vi "Save Icon.vi"(8 "error in (no error)":errorcluster, 10 "path":path, 11 "vi ref":refnum<vi>) -> (0 "error out":errorcluster, 2 "path out":path, 3 "reference out":refnum<vi>)   [LabVIEW 2014, in "lvprj2html.lvlib"]
uses:
  lvprj2html.lvlib
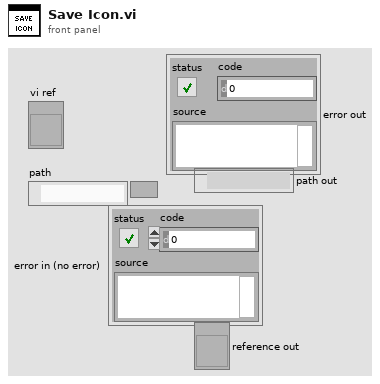
[diagram p1: front panel]
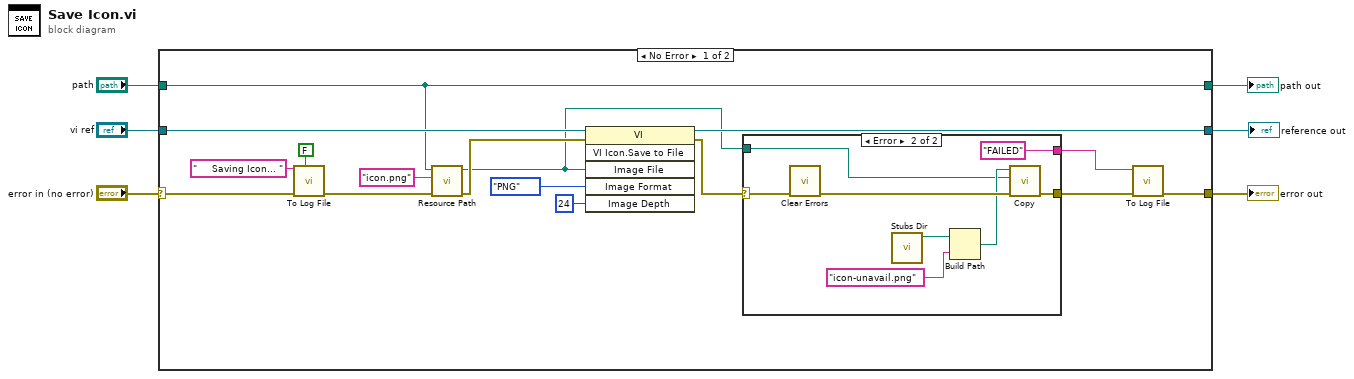
[diagram p0: block diagram]
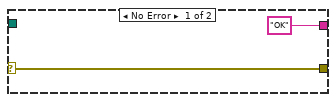
[diagram p2: hidden frame]
diagram:
  n1 = case shown="No Error" "error in (no error)" {
    selector: "error in (no error)" -> [w8 w35]
    tunnel: "vi ref" -> [w22 w34]
    tunnel: "path" -> [w7 w33]
    tunnel: [w17 w34] -> w4
    tunnel: [w9 w35] -> w3
    tunnel: [w7 w33] -> w1
    frame No Error {
      n2 = call "To Log File.vi"("new line"=FALSE, "error in (no error)"=w8, "string"="     Saving Icon... " ("format string")) -> ("error out"=w14:errorcluster)  [unwired: 8 in]
      n3 = call "Resource Path.vi"("error in (no error)"=w14, "resource file name"="icon.png", "data dir"=w7) -> ("error out"=w18:errorcluster, "path"=w10:path)  [unwired: 7 in]
      n4 = invoke class="VI" method="VI Icon.Save to File"(reference=w22, error in=w18, "Image File"=w10, "Image Format"=enum32{"PNG", "JPEG", "GIF", "BMP"}."PNG", "Image Depth"=24) -> (reference out=w17:refnum<vi>, error out=w11:errorcluster)  [unwired: 1 in, 4 out]
      n5 = case shown="Error" w11 {
        selector: w11 -> [w24 w32]
        tunnel: [w24 w25] -> w12
        tunnel: ["OK" ("string") "FAILED" ("string")] -> w13
        tunnel: w10 -> [_ w26]
        frame No Error {
        }
        frame Error {
          n6 = call <vilib>:"Clear Errors.vi"("error in (no error)"=w32) -> ("error out"=w28:errorcluster)  [unwired: 5 in, 1 out]
          n7 = call "Stubs Dir.vi"() -> ("path"=w29:path)  [unwired: 11 in]
          n8 = Build Path(base path=w29, name or relative path="icon-unavail.png") -> (appended path=w27:path)
          n9 = call "Copy.vi"("error in (no error)"=w28, "dst"=w26, "src"=w27) -> ("error out"=w25:errorcluster)  [unwired: 8 in]
        }
      }
      n10 = call "To Log File.vi"("error in (no error)"=w12, "string"=w13) -> ("error out"=w9:errorcluster)  [unwired: 9 in]
    }
    frame Error {
    }
  }
  "error out" <- w3
  "reference out" <- w4
  "path out" <- w1
